vi "Get 3d point cloud.vi"(6 "Sensor Yaw":sgl, 7 "Depth Scalar":dbl=185.63 format="%#_13g", 8 "Floor threshold":dbl=6.0 format="%#_13g", 9 "Sensor height":dbl, 10 "Elevation Angle":i32(slide) scale=-27.0..27.0, 11 "Depth Array":i16[][](array[numeric])) -> (3 "Points":cluster{"Data":sgl, "Data":sgl, "Data":sgl}[](array[cluster]))   [LabVIEW 2014]
uses:
  <vilib>/Analysis/coordinate.llb/3D Coordinate Conversion (Scalar).vi
  <vilib>/Analysis/NI_AALPro.lvlib
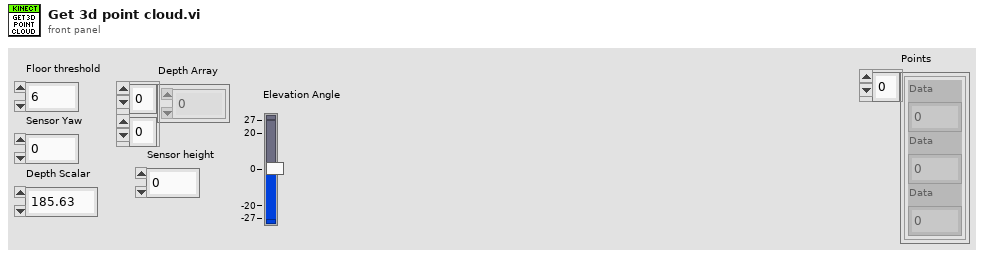
[diagram p1: front panel]
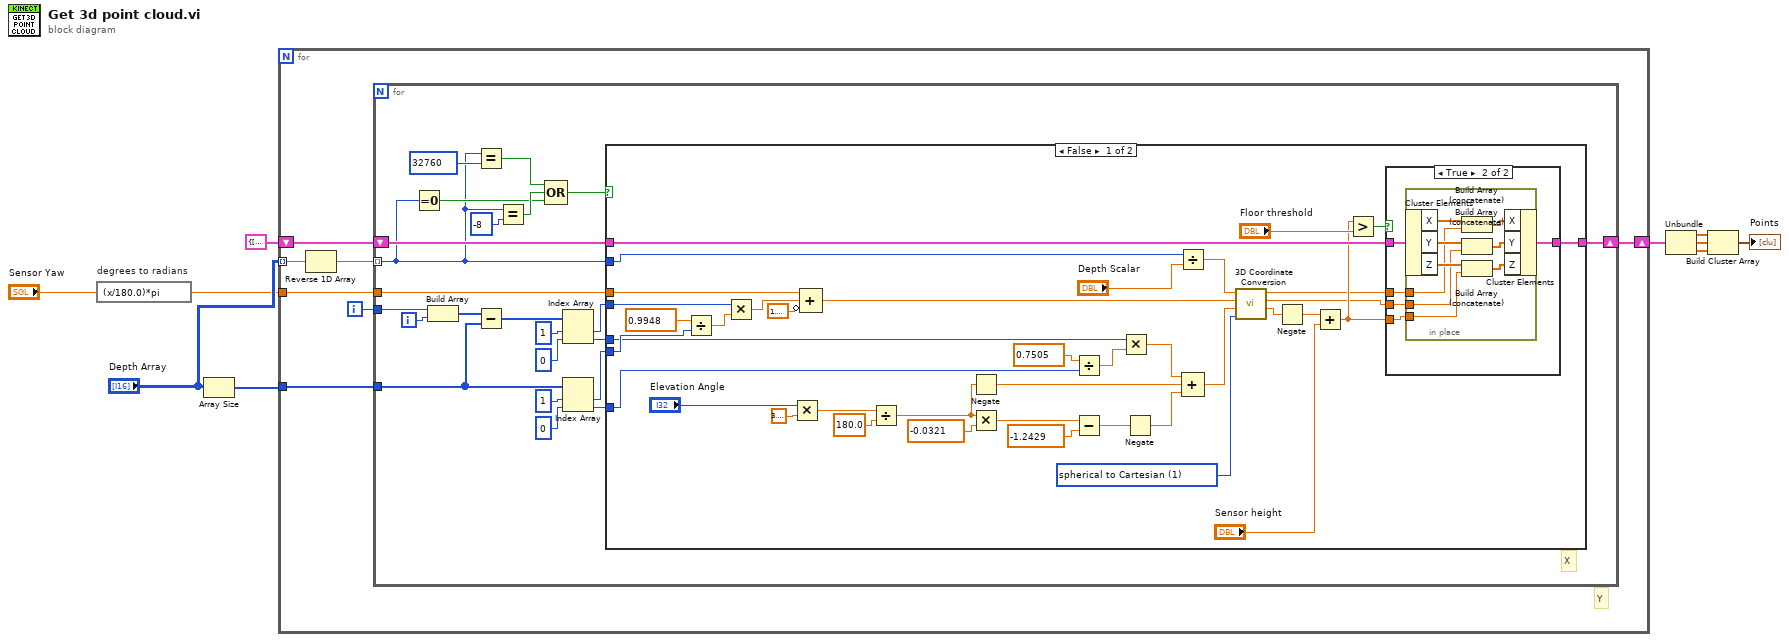
[diagram p0: block diagram]
diagram:
  n1 = expression code="(x/180.0)*pi" "degrees to radians"("Sensor Yaw") -> (w1:sgl)
  n2 = Array Size(array="Depth Array") -> (size(s)=w9:i32[])
  n3 = for {
    tunnel: "Depth Array" -> [w12] mode=indexing
    shift-right: [w15] -> w3
    shift-left: cluster{"X":sgl[], "Y":sgl[], "Z":sgl[]} {"X"=[], "Y"=[], "Z"=[]} -> [w16]
    tunnel: w9 -> [w14]
    tunnel: w1 -> [w11]
    i -> [w17]
    # "Y"
    n4 = Reverse 1D Array(array=w12) -> (reversed array=w13:i16[])
    n5 = for {
      tunnel: w13 -> [w22] mode=indexing
      tunnel: w17 -> [w32]
      shift-right: [w37] -> w15
      shift-left: w16 -> [w38]
      tunnel: w14 -> [w27]
      tunnel: w11 -> [w18]
      i -> [w21]
      # "X"
      n6 = Equal To 0?(x=w22) -> (x = 0?=w34:bool)
      n7 = Build Array(w32, w21) -> (w31:i32[])
      n8 = Equal?(x=w22, y=i16 32760) -> (x = y?=w35:bool)
      n9 = Subtract(x=w31, y=w27) -> (x-y=w28:i32[])
      n10 = Equal?(x=w22, y=i16 -8) -> (x = y?=w36:bool)
      n11 = Compound Arithmetic op=OR(w35, w36, w34) -> (w33:bool)
      n12 = Index Array(array=w28, index #1=1 ("index"), index #2=0 ("index")) -> (element #1=w30:i32, element #2=w29:i32)
      n13 = Index Array(array=w27, index #1=1 ("index"), index #2=0 ("index")) -> (element #1=w26:i32, element #2=w25:i32)
      n14 = case shown="False" w33 {
        tunnel: w38 -> [w79 w95]
        tunnel: [w78 w95] -> w37
        tunnel: w30 -> [w72 _]
        tunnel: w29 -> [w70 _]
        tunnel: w26 -> [w74 _]
        tunnel: w25 -> [w76 _]
        tunnel: w22 -> [w64 _]
        tunnel: w18 -> [w41 _]
        frame False {
          w63 = u16 1 items=["Cartesian to spherical", "spherical to Cartesian", "Cartesian to cylindrical", "cylindrical to Cartesian", "spherical to cylindrical", "cylindrical to spherical"] ("conversion type")
          n15 = Divide(x=0.9948, y=w74) -> (x/y=w73:dbl)
          n16 = Multiply(x=w72, y=w73) -> (x*y=w44:dbl)
          n17 = Multiply(x="Elevation Angle", y=3.141592653589793) -> (x*y=w67:dbl)
          n18 = Compound Arithmetic op=ADD(w41, w44, invert 1.5707963267948966) -> (w42:dbl)
          n19 = Divide(x=w67, y=180.0) -> (x/y=w53:dbl)
          n20 = Negate(x=w53) -> (-x=w52:dbl)
          n21 = Multiply(x=w53, y=-0.0321) -> (x*y=w57:dbl)
          n22 = Divide(x=0.7505, y=w76) -> (x/y=w71:dbl)
          n23 = Subtract(x=w57, y=-1.2429) -> (x-y=w55:dbl)
          n24 = Multiply(x=w70, y=w71) -> (x*y=w69:dbl)
          n25 = Negate(x=w55) -> (-x=w54:dbl)
          n26 = Divide(x=w64, y="Depth Scalar") -> (x/y=w62:dbl)
          n27 = Compound Arithmetic op=ADD(w69, w52, w54) -> (w61:dbl)
          n28 = call-poly <vilib>:"3D Coordinate Conversion.vi"("conversion type"=w63, "axis 3"=w61, "axis 2"=w42, "axis 1"=w62) -> ("axis 3 out"=w59:dbl, "axis 2 out"=w45:dbl, "axis 1 out"=w46:dbl)  [unwired: 4 in, 1 out]
          n29 = Negate(x=w59) -> (-x=w51:dbl)
          n30 = Add(x=w51, y="Sensor height") -> (x+y=w47:dbl)
          n31 = Greater?(x=w47, y="Floor threshold") -> (0:w50:bool)
          n32 = case shown="True" w50 {
            tunnel: w79 -> [w80 w85]
            tunnel: [w80 w84] -> w78
            tunnel: w46 -> [_ w83]
            tunnel: w45 -> [_ w82]
            tunnel: w47 -> [_ w81]
            frame False {
            }
            frame True {
              n33 = in-place {
                in-place-border: w83 -> [w88]
                in-place-border: w82 -> [w87]
                in-place-border: w81 -> [w86]
                n34 = in-place-cluster #1(w85) -> ("X"=w89:sgl[], "Y"=w90:sgl[], "Z"=w92:sgl[])
                n35 = Build Array (concatenate)(w89, w88) -> (w94:dbl[])
                n36 = Build Array (concatenate)(w90, w87) -> (w93:dbl[])
                n37 = Build Array (concatenate)(w92, w86) -> (w91:dbl[])
                n38 = in-place-cluster #1("X"=w94, "Y"=w93, "Z"=w91) -> (w84:cluster{"X":sgl[], "Y":sgl[], "Z":sgl[]})
              }
            }
          }
        }
        frame True {
        }
      }
    }
  }
  n39 = Unbundle(w3) -> ("X"=w7:sgl[], "Y"=w6:sgl[], "Z"=w5:sgl[])
  n40 = Build Cluster Array(w7, w6, w5) -> (→"Points":cluster{"Data":sgl, "Data":sgl, "Data":sgl}[])
